vi "SendStopUE.vi"(8 "Error In":errorcluster) -> (0 "Error Out":errorcluster)   [LabVIEW 2017, in "StopUE.lvlib"]
uses:
  StopUE.lvlib
  States_FGV.ctl
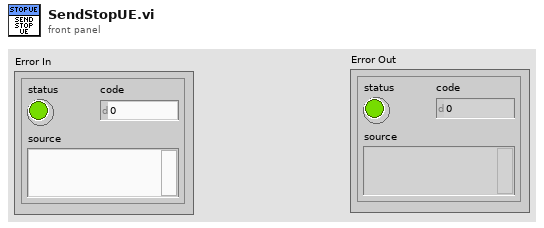
[diagram p1: front panel]
types:
  T1 = typedef "StopUE.lvlib/States_FGV.ctl" = enum16{"Get", "Shutdown", "Initialize"}
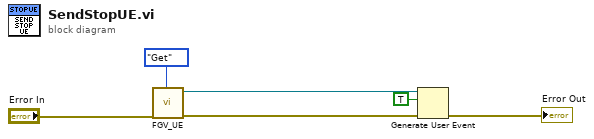
[diagram p0: block diagram]
diagram:
  n1 = call "FGV_UE.vi"("State"=States_FGV."Get", "Error In"="Error In") -> ("Error Out"=w3:errorcluster, "STOP"=w4:refnum<user-event>)  [unwired: 8 in]
  n2 = Generate User Event(user event=w4, event data cluster=TRUE ("event data"), error in=w3) -> (error out=→"Error Out":errorcluster)  [unwired: 1 in, 1 out]
